vi "CH_LM Config Measurement Delivery Mode.vi"(0 "Meter Index":i32, 2 "Delivery Mode":T1, 5 "error in (no error)":errorcluster, 7 "Timeout / ms (3000)":i32=3000, 8 "Action (query)":bool, 9 "Lock Timeout / ms (1000)":i32=1000) -> (11 "Lock timed out":bool, 14 "Meter Index":i32, 16 "Delivery Mode":T1, 19 "error out":errorcluster)   [LabVIEW 2012, in "CH_LM.lvlib"]
doc: "This command will select if data delivery for thermopile or optical probes is presented in a continuous stream of sampled data records or simply the last available data record.\n\n<B>Attention:</B> If this command is issued while data collection is enabled the setting will not take effect until the next data collection cycle begins."
uses:
  CH_LM.lvlib
  CH_LM Measurement Delivery Mode.ctl
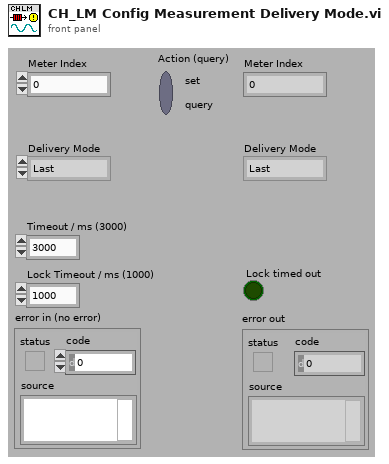
[diagram p1: front panel]
types:
  T1 = typedef "CH_LM.lvlib/CH_LM Measurement Delivery Mode.ctl" = enum16{"Last", "Stream"}
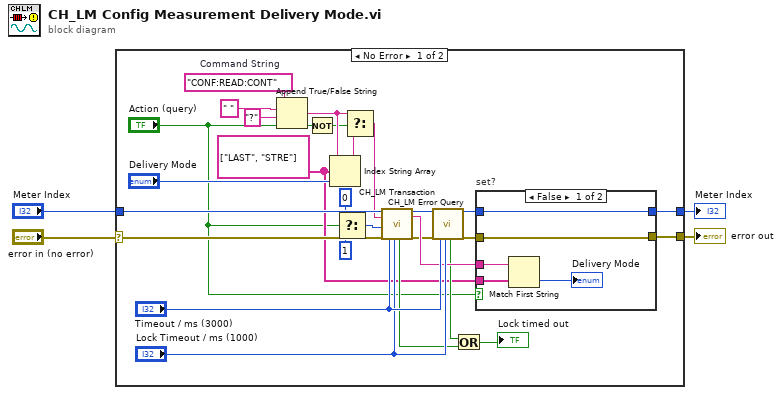
[diagram p0: block diagram]
diagram:
  n1 = case shown="No Error" "error in (no error)" {
    selector: "error in (no error)" -> [w31 w40]
    tunnel: [w29 w40] -> w4
    tunnel: "Meter Index" -> [w30 w39]
    tunnel: [w28 w39] -> w1
    frame No Error {
      w10 = string[] ["LAST", "STRE"] ("string array")
      w25 = "CONF:READ:CONT"  # Command String
      n2 = Append True/False String(1:"Action (query)", 2:"?" ("true string"), 3:" ", 4:w25) -> (0:w9:string)
      n3 = Not(x="Action (query)") -> (.not. x?=w5:bool)
      n4 = Index String Array(1:"Delivery Mode", 2:w10, 3:w9) -> (0:w7:string)
      n5 = Select(t=0, s="Action (query)", f=1 ("NofStrings (-1:all)")) -> (s? t:f=w21:i32)
      n6 = Select(t=w9, s=w5, f=w7) -> (s? t:f=w8:string)
      n7 = call "CH_LM Transaction.vi"("Meter Index"=w30, "Command String"=w8, "NofStrings (-1:all)"=w21, "error in (no error)"=w31, "Timeout / ms (3000)"="Timeout / ms (3000)", "Lock Timeout / ms (1000)"="Lock Timeout / ms (1000)") -> ("Lock timed out"=w14:bool, "Meter Index"=w19:i32, "Response"=w24:string, "error out"=w17:errorcluster)  [unwired: 10 out]
      n8 = call "CH_LM Error Query.vi"("Meter Index"=w19, "error in (no error)"=w17, "Timeout / ms (3000)"="Timeout / ms (3000)", "Lock Timeout / ms (1000)"="Lock Timeout / ms (1000)") -> ("Lock timed out"=w15:bool, "Meter Index"=w18:i32, "error out"=w16:errorcluster)  [unwired: 13 out]
      n9 = Or(x=w15, y=w14) -> (x .or. y?=→"Lock timed out":bool)
      n10 = case "set?" shown="False" "Action (query)" {
        tunnel: w24 -> [w35 _]
        tunnel: w16 -> [w34 w38]
        tunnel: [w34 w38] -> w29
        tunnel: w18 -> [w36 w37]
        tunnel: [w36 w37] -> w28
        tunnel: w10 -> [w32 _]
        frame False {
          n11 = Match First String(2:w32, 3:w35) -> (0:→"Delivery Mode":i32)  [unwired: 1 out]
        }
        frame True {
        }
      }
    }
    frame Error {
    }
  }
  "error out" <- w4
  "Meter Index" <- w1
